vi "NewGame.vi"(7 "GameType (ChildObject)":refnum<class "Game.lvclass">, 8 "error in (no error)":errorcluster, 11 "FPGA_ref":T1) -> (0 "error out":errorcluster, 3 "Game out":refnum<class "Game.lvclass">)   [LabVIEW 2019, in "RT_Game.lvlib" / "Game.lvclass"]
uses:
  Game.lvclass
  FPGA_Interface.ctl
  RT_Sprite/RT_Sprite.lvclass
  Game.lvclass/Game.ctl
  <vilib>/Utility/error.llb/Error Cluster From Error Code.vi
  <vilib>/rvi/errors/niLvFpgaAdjustHostInterfaceError.vi
  <vilib>/rvi/interface/common/niFpgaWaitOnOcc.vi
  <vilib>/rvi/interface/nirviReadWriteControl/nirviReadWriteControl.xnode
  FPGA Bitfiles/myriogameconsole_FPGATarget_Main_ntsPRcBZGxk.lvbitx
  <vilib>/rvi/interface/nirviMethod/nirviMethod.xnode
  NiFpgaLv.dll
  <vilib>/FPGAPlugInAG/myRIO-1900/niLvFpga_ConfigureFifo_myRIO-1900.vi
  <vilib>/rvi/errors/niLvFpgaMergeErrorWithErrorCode.vi
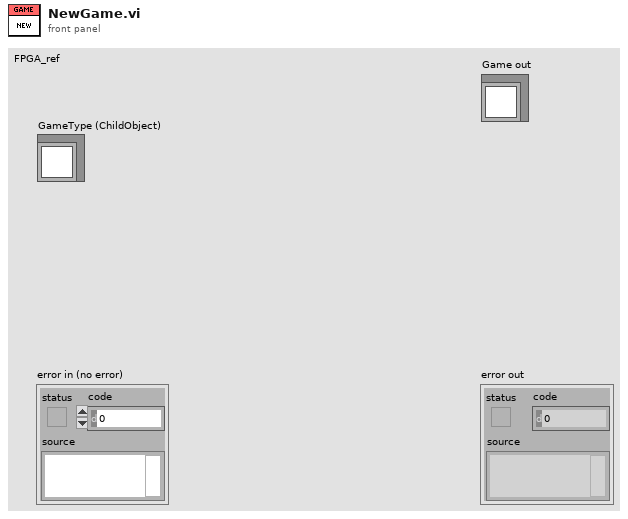
[diagram p1: front panel]
types:
  T1 = typedef "FPGA_Interface.ctl" = refnum<k20>
  T2 = cluster{"[0]":refnum<class "RT_Sprite.lvclass">, "[1]":refnum<class "RT_Sprite.lvclass">, "[2]":refnum<class "RT_Sprite.lvclass">}
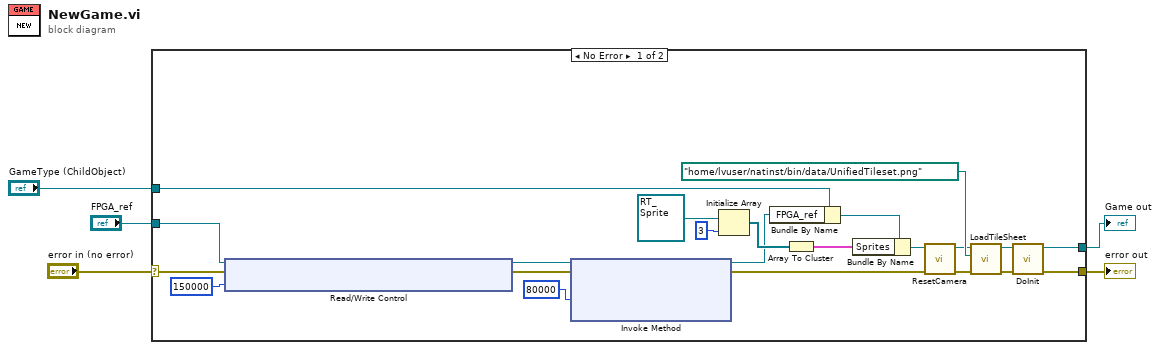
[diagram p0: block diagram]
diagram:
  n1 = case shown="No Error" "error in (no error)" {
    selector: "error in (no error)" -> [w12 w29]
    tunnel: [w25 w29] -> w4
    tunnel: [w24 w28] -> w3
    tunnel: "GameType (ChildObject)" -> [w13 w28]
    tunnel: "FPGA_ref" -> [w26 _]
    frame No Error {
      n2 = xnode "Read/Write Control"("FPGA VI Reference In"=w26, "error in"=w12, "FadeRate"=u32 150000) -> ("FPGA VI Reference Out"=w18:T1, "error out"=w23:errorcluster)
      n3 = xnode "Invoke Method"("FPGA VI Reference In"=w18, "error in"=w23, "Requested Depth"=u32 80000) -> ("FPGA VI Reference Out"=w16:T1, "error out"=w17:errorcluster)  [unwired: 1 out]
      n4 = Initialize Array(refnum<class "RT_Sprite.lvclass"> refnum ("RT_Game.lvlib:RT_Sprite.lvclass"), 3 ("dimension size")) -> (w19:refnum<class "RT_Sprite.lvclass">[])
      n5 = Bundle By Name(cluster=w13, "FPGA_ref"=w16) -> (w20:refnum<class "Game.lvclass">)
      n6 = Array To Cluster(array=w19) -> (cluster=w11:T2)
      n7 = Bundle By Name(cluster=w20, "Sprites"=w11) -> (w9:refnum<class "Game.lvclass">)
      n8 = call "ResetCamera.vi"("error in (no error)"=w17, "Game in"=w9) -> ("error out"=w10:errorcluster, "Game out"=w8:refnum<class "Game.lvclass">)  [unwired: 8 in]
      n9 = call "LoadTileSheet.vi"("error in (no error)"=w10, "Tile Path"=path "/home/lvuser/natinst/bin/data/UnifiedTileset.png", "Game in"=w8) -> ("error out"=w6:errorcluster, "Game out"=w7:refnum<class "Game.lvclass">)  [unwired: 7 in]
      n10 = call-dynamic "DoInit.vi"("error in (no error)"=w6, "Game in"=w7) -> ("error out"=w25:errorcluster, "Game out"=w24:refnum<class "Game.lvclass">)  [unwired: 8 in]
    }
    frame Error {
    }
  }
  "error out" <- w4
  "Game out" <- w3
